vi "Load_16bit_Array.vi"(4 "Load in PCO Format":bool=TRUE, 5 "Load Array":bool=TRUE, 6 "Use Name and Number":bool, 7 "Take Full Path":bool=TRUE, 8 "error in (no error)":errorcluster, 9 "Path":path=path "\\\\Walnuss\\Silverbrick/Lab/Stefan/Data/041108/C63/s_0001.b16", 10 "Name":string, 11 "Number":i32) -> (0 "error out":errorcluster, 3 "Fluorescence Image":dbl[][](graph))   [LabVIEW 2010]
panel:
  in  "Number for Array":i32
  in  "File Options":T1={"Read Raw File"=0, "File Data Type"=4, "Offset to Data"=0, "Use Min Max"=enum."Don't use min max", "Optional Min Value"=0.0, "Optional Max Value"=0.0, "Byte Order"=enum."Big endian (Motorola)"} {"Optional Max Value" format="%.2f"; "Optional Min Value" format="%.2f"; "File Data Type" items=["1 bit", "2 bits", "4 bits", "8 bits", "16 bits (unsigned)", "16 bits (signed)", "16 bits (RGB chunky)", "24 bits (RGB chunky)", "24 bits (RGB planar)", "32 bits (unsigned)", "32 bits (signed)", "32 bits (RGB chunky)", "32 bits (float)", "48 bits (Complex 2x24 int)", "64 bits (Complex 2x32 float)", "32 bits (HSL)"]; "Read Raw File" items=["Don't Read Raw File ", "Read Raw File"]}
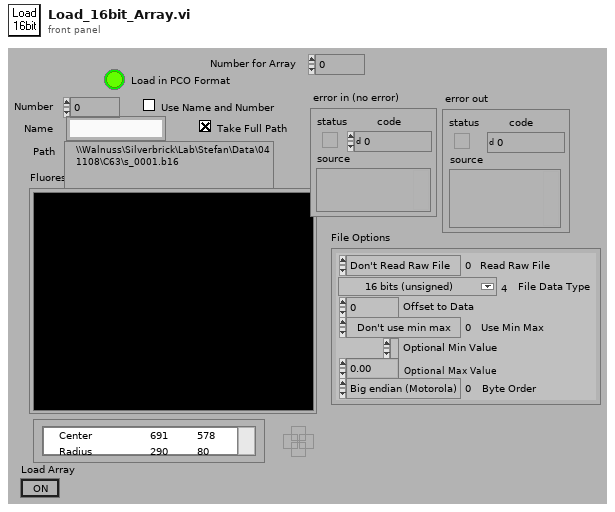
[diagram p1: front panel]
types:
  T1 = cluster{"Read Raw File":i32, "File Data Type":u32, "Offset to Data":i32, "Use Min Max":enum32{"Don't use min max", "Use file values", "Use optional values"}, "Optional Min Value":sgl, "Optional Max Value":sgl, "Byte Order":enum32{"Big endian (Motorola)", "Little endian (Intel)"}}
  T2 = enum16{"read/write", "read-only", "write-only", "write-only (truncate)"}
  T3 = typedef "Image Type" = u32
  T4 = typedef "IMAQ Image.ctl" = refnum<image>
  T5 = enum16{"open", "open or create", "create or replace", "create", "open (read only)"}
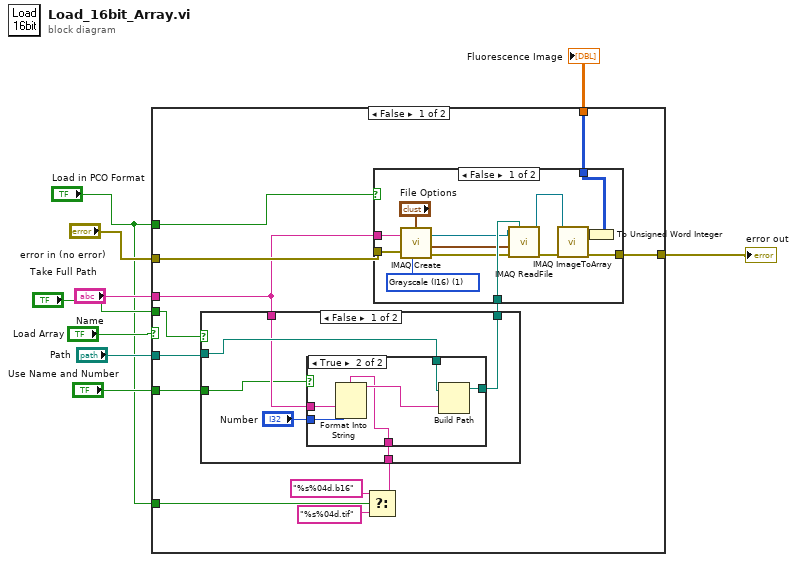
[diagram p0: block diagram]
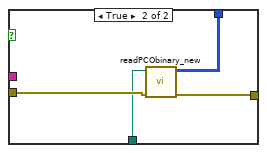
[diagram p2: hidden frame]
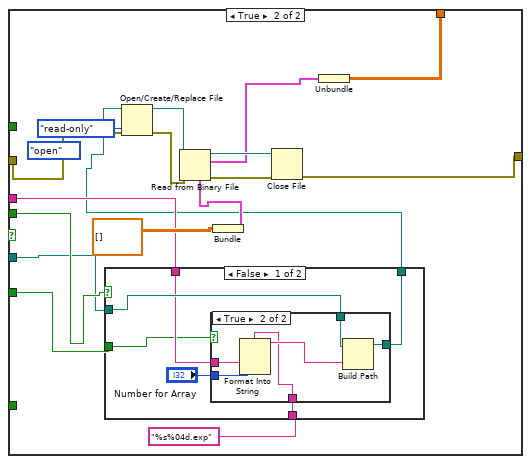
[diagram p5: hidden frame]
diagram:
  n1 = case shown="False" "Load Array" {
    tunnel: "Load in PCO Format" -> [w22 _]
    tunnel: [w21 w69] -> w9
    tunnel: [w20 w66] -> w8
    tunnel: "error in (no error)" -> [w19 w55]
    tunnel: "Path" -> [w14 w60]
    tunnel: "Name" -> [w13 w58]
    tunnel: "Use Name and Number" -> [w12 w61]
    tunnel: "Take Full Path" -> [w11 w62]
    tunnel: "Load in PCO Format" -> [w10 _]
    frame False {
      n2 = Select(t="%s%04d.b16" ("Format String"), s=w10, f="%s%04d.tif" ("Format String")) -> (s? t:f=w15:string)
      n3 = case shown="False" w11 {
        tunnel: [w42 w52] -> w18
        tunnel: w14 -> [w43 w52]
        tunnel: w13 -> [w41 _]
        tunnel: w15 -> [w40 _]
        tunnel: w12 -> [w39 _]
        frame False {
          n4 = case shown="True" w39 {
            tunnel: "Number" -> [_ w51]
            tunnel: w43 -> [w45 w49]
            tunnel: [w45 w50] -> w42
            tunnel: w41 -> [_ w47]
            tunnel: w40 -> [_ w46]
            frame False {
            }
            frame True {
              n5 = Format Into String(format string=w46, w47, w51) -> (resulting string=w48:string)  [unwired: 2 in, 1 out]
              n6 = Build Path(base path=w49, name or relative path=w48) -> (appended path=w50:path)
            }
          }
        }
        frame True {
        }
      }
      n7 = case shown="False" w22 {
        tunnel: w18 -> [w34 w36]
        tunnel: w13 -> [w29 _]
        tunnel: [w28 w37] -> w21
        tunnel: w19 -> [w27 w38]
        tunnel: [w23 w35] -> w20
        frame False {
          w25 = T3 1 items=["Grayscale (U8)", "Grayscale (I16)", "Grayscale (SGL)", "Complex (CSG)", "RGB (U32)", "HSL (U32)", "RGB (U64)", "Grayscale (U16)"] ("Image Type")
          n8 = call "IMAQ Create"("Image Name"=w29, "Image Type"=w25, "error in (no error)"=w27) -> ("New Image"=w26:T4, "error out"=w33:errorcluster)  [unwired: 2 in]
          n9 = call "IMAQ ReadFile"("File Path"=w34, "error in (no error)"=w33, "File Options"="File Options", "Image"=w26) -> ("error out"=w31:errorcluster, "Image Out"=w30:T4)  [unwired: 3 in, 3 out]
          n10 = call "IMAQ ImageToArray"("error in (no error)"=w31, "Image"=w30) -> ("error out"=w28:errorcluster, "Image Pixels (I16)"=w24:i16[][])  [unwired: 2 in, 3 out]
          n11 = To Unsigned Word Integer(number=w24) -> (unsigned 16bit integer=w23:u16[][])
        }
        frame True {
          n12 = call "readPCObinary_new.vi"("error in (no error)"=w38, "Image Path"=w36) -> ("error out"=w37:errorcluster, "Image"=w35:u16[][])  [unwired: 8 in]
        }
      }
    }
    frame True {
      (unwired) T5."open" ("function (open:0)")
      n13 = case shown="False" w62 {
        tunnel: [w73 w83] -> w57
        tunnel: w60 -> [w74 w83]
        tunnel: w58 -> [w72 _]
        tunnel: "%s%04d.exp" ("Format String") -> [w71 _]
        tunnel: w61 -> [w70 _]
        frame False {
          n14 = case shown="True" w70 {
            tunnel: "Number for Array" -> [_ w82]
            tunnel: w74 -> [w76 w80]
            tunnel: [w76 w81] -> w73
            tunnel: w72 -> [_ w78]
            tunnel: w71 -> [_ w77]
            frame False {
            }
            frame True {
              n15 = Format Into String(format string=w77, w78, w82) -> (resulting string=w79:string)  [unwired: 2 in, 1 out]
              n16 = Build Path(base path=w80, name or relative path=w79) -> (appended path=w81:path)
            }
          }
        }
        frame True {
        }
      }
      n17 = Open/Create/Replace File(file path (use dialog)=w57, error in=w55, access (0:read/write)=T2."read-only" ("open mode (0)")) -> (refnum out=w53:refnum<file>, error out=w54:errorcluster)  [unwired: 3 in, 1 out]
      n18 = Bundle("element"=dbl[][] []) -> (w63:cluster{"element":dbl[][]})  [unwired: 1 in]
      n19 = Read from Binary File(5:w63, 8:w54, 11:w53) -> (0:w64:errorcluster, 2:w67:cluster{"element":dbl[][]}, 3:w68:refnum<file>)  [unwired: 3 in, 1 out]
      n20 = Close File(refnum=w68, error in=w64) -> (error out=w69:errorcluster)  [unwired: 1 out]
      n21 = Unbundle(w67) -> ("element"=w66:dbl[][])
    }
  }
  "error out" <- w9
  "Fluorescence Image" <- w8
